vi "libssh2_init_custom.vi"(8 "error in (no error)":errorcluster, 10 "flags (0 = none)":T1 items=["No Crypto"=1], 11 "path (use built-in)":path) -> (0 "error out":errorcluster)   [LabVIEW 2017, in "libssh2.lvlib"]
doc: "Initialize libssh2 with a custom build of libssh2."
uses:
  libssh2.lvlib
  libssh2_init_flags.ctl
  Global Settings.vi
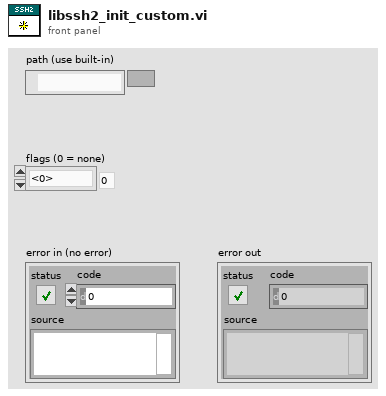
[diagram p1: front panel]
types:
  T1 = typedef "libssh2.lvlib/libssh2_init_flags.ctl" = i32
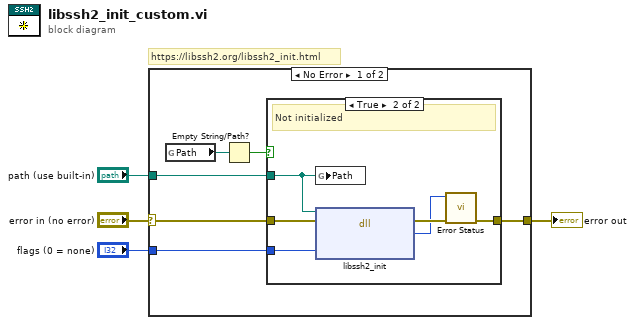
[diagram p0: block diagram]
diagram:
  # "https://libssh2.org/libssh2_init.html"
  n1 = case shown="No Error" "error in (no error)" {
    selector: "error in (no error)" -> [w9 w18]
    tunnel: [w10 w18] -> w4
    tunnel: "path (use built-in)" -> [w8 _]
    tunnel: "flags (0 = none)" -> [w5 _]
    frame No Error {
      n2 = global read "Global Settings.vi" "Path"() -> (w6:path)
      n3 = Empty String/Path?(string/path=w6) -> (empty?=w7:bool)
      n4 = case shown="True" w7 {
        tunnel: [w11 w14] -> w10
        tunnel: w9 -> [w11 w16]
        tunnel: w8 -> [_ w15]
        tunnel: w5 -> [_ w12]
        frame False {
          # "Already initialized"
        }
        frame True {
          # "Not initialized"
          n5 = global write "Global Settings.vi" "Path"(w15) -> ()
          n6 = dll-call lib="?" fn="libssh2_init"(path in=w15, error in=w16, "flags"=w12) -> (error out=w17:errorcluster, "return value"=w13:i32)  [unwired: 2 in, 1 out]
          n7 = call "Error Status.vi"("error in (no error)"=w17, "return value"=w13) -> ("error out"=w14:errorcluster)  [unwired: 8 in, 1 out]
        }
      }
    }
    frame Error {
    }
  }
  "error out" <- w4
